vi "GetAttribute2.vi"(0 "reference in":refnum<class "G#SubSubClass2.lvclass">, 5 "error in (no error)":errorcluster) -> (12 "Locked":bool, 14 "reference out":refnum<class "G#SubSubClass2.lvclass">, 15 "Base class.Base class.Numeric":dbl, 16 "Base class.SubAttribute":dbl, 17 "Base class.Base class.Array":dbl[](array[numeric]), 18 "SubSubAttribute":dbl, 19 "error out":errorcluster)   [LabVIEW 2010, in "G#SubSubClass2.lvclass"]
uses:
  G#SubSubClass2.lvclass
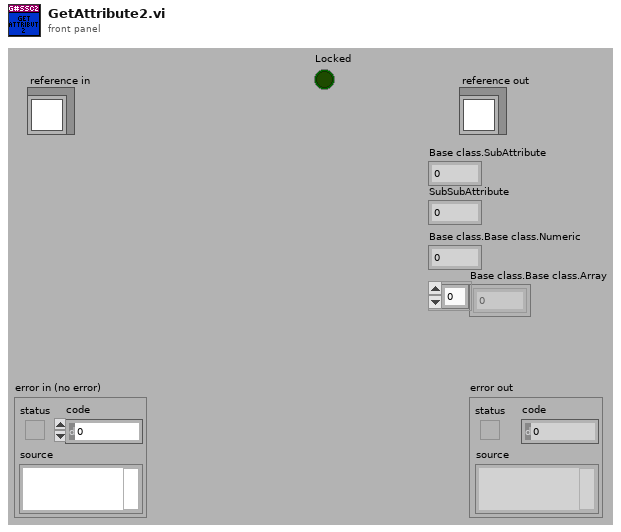
[diagram p1: front panel]
types:
  T1 = typedef "G#SubSubClass2.lvclass/ObjectAttributes.ctl" = cluster{"Base class":T2, "SubSubAttribute":dbl}
  T2 = typedef "G#SubClass2.lvclass/ObjectAttributes.ctl" = cluster{"Base class":T3, "SubAttribute":dbl}
  T3 = typedef "G#BaseClass2.lvclass/ObjectAttributes.ctl" = cluster{"Numeric":dbl, "Array":dbl[]}
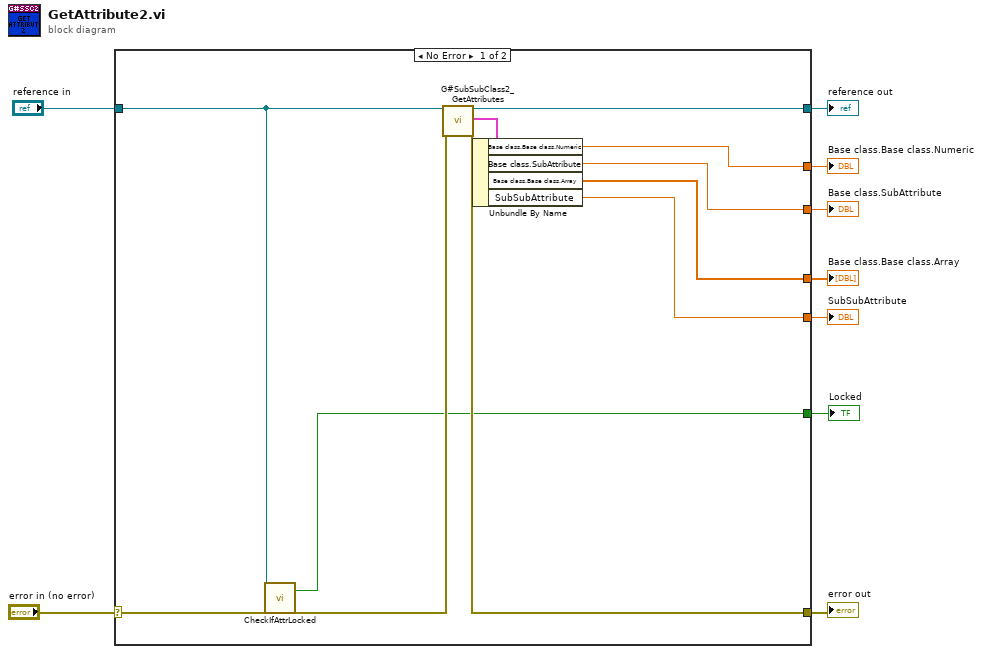
[diagram p0: block diagram]
diagram:
  n1 = case shown="No Error" "error in (no error)" {
    selector: "error in (no error)" -> [w13 w22]
    tunnel: [w19 w22] -> w8
    tunnel: [w18 w21] -> w6
    tunnel: "reference in" -> [w12 w21]
    tunnel: [w17 _] -> w5
    tunnel: [w16 _] -> w4
    tunnel: [w15 _] -> w3
    tunnel: [w14 _] -> w2
    tunnel: [w10 _] -> w1
    frame No Error {
      n2 = call-dynamic "CheckIfAttrLocked.vi"("reference in"=w12, "error in (no error)"=w13) -> ("locked"=w10:bool, "error out"=w11:errorcluster)  [unwired: 15 in, 1 out]
      n3 = call "G#SubSubClass2_GetAttributes.vi"("reference in"=w12, "error in (no error)"=w11) -> ("reference out"=w18:refnum<class "G#SubSubClass2.lvclass">, "attributes"=w20:T1, "error out"=w19:errorcluster)  [unwired: 14 in, 1 out]
      n4 = Unbundle By Name(w20) -> ("Base class.Base class.Numeric"=w17:dbl, "Base class.SubAttribute"=w16:dbl, "Base class.Base class.Array"=w15:dbl[], "SubSubAttribute"=w14:dbl)
    }
    frame Error {
    }
  }
  "error out" <- w8
  "reference out" <- w6
  "Base class.SubAttribute" <- w4
  "Base class.Base class.Array" <- w3
  "Base class.Base class.Numeric" <- w5
  "SubSubAttribute" <- w2
  "Locked" <- w1
